vi "ParseBoolChannel.vi"(11 "Input":string) -> (3 "Array":bool[](array[boolean]))   [LabVIEW 2019]
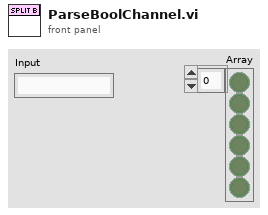
[diagram p1: front panel]
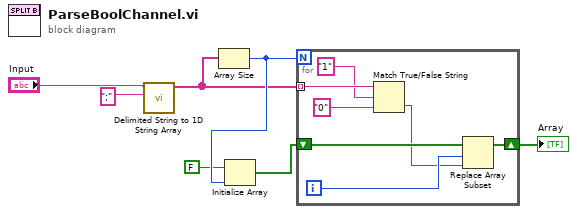
[diagram p0: block diagram]
diagram:
  n1 = call <vilib>:"Delimited String to 1D String Array.vi"("delimiter"=";" ("search string/char (-)"), "delimited string"="Input") -> ("string array"=w4:string[])  [unwired: 9 in]
  n2 = Array Size(array=w4) -> (size(s)=w5:i32)
  n3 = Initialize Array(FALSE, w5) -> (w2:bool[])
  n4 = for {
    N: w5 -> [_]
    tunnel: w4 -> [w11] mode=indexing
    shift-right: [w13] -> w3
    shift-left: w2 -> [w12]
    i -> [w14]
    n5 = Match True/False String(2:"0" ("false string"), 3:"1" ("true string"), 4:w11) -> (0:w10:bool)  [unwired: 1 out]
    n6 = Replace Array Subset(array=w12, new element=w10, index=w14) -> (w13:bool[])
  }
  "Array" <- w3
